vi "Barkod Tarayici.vi"() -> ()   [LabVIEW 2017]
uses:
  <vilib>/userdefined/High Color/IMAQdx.ctl
  <vilib>/Utility/file.llb/Read Delimited Spreadsheet (string).vi
  <vilib>/vision/driver/NI_Vision_Acquisition_Software.lvlib
  <vilib>/vision/NI_Vision_Development_Module.lvlib
panel:
  out "Kullanım":string[](array[string])
  out "İlaç İsmi":string[](array[string])
  out "Barkod":string[](array[string])
  out "all rows":string[][](array[string])
  in  "İlaç Listesi":path
  in  "Listeyi Yükle":bool
  out "İlaç Bilgisi":string
  out "Barkod Bulundu":bool
  out "error out 3":errorcluster
  out "Barkod Numarası":string
  in  "Aranacak Barkod Türleri":u32[](array[ring])=[6, 4] items=["Reserved", "Codabar", "Code 39", "Code 93", "Code 128", "EAN 8", "EAN 13", "Interleaved 2 of 5", "MSI", "UPCA", "Pharmacode", "RSS Limited"]
  out "error out 2":errorcluster
  out "error out":errorcluster
  out "Barkod":T1(array[cluster]) {"Confidence Level" format="%.2f"; "Barcode Type" items=["Reserved", "Codabar", "Code 39", "Code 93", "Code 128", "EAN 8", "EAN 13", "Interleaved 2 of 5", "MSI", "UPCA", "Pharmacode", "RSS Limited"]; "Bounding Box"."y" format="%.2f"; "Bounding Box"."x" format="%.2f"}
  out "Görüntü":T2(plugin-control)
  in  "Durdur":bool
  in  "Kamera Kaynağı Seçiniz":T3
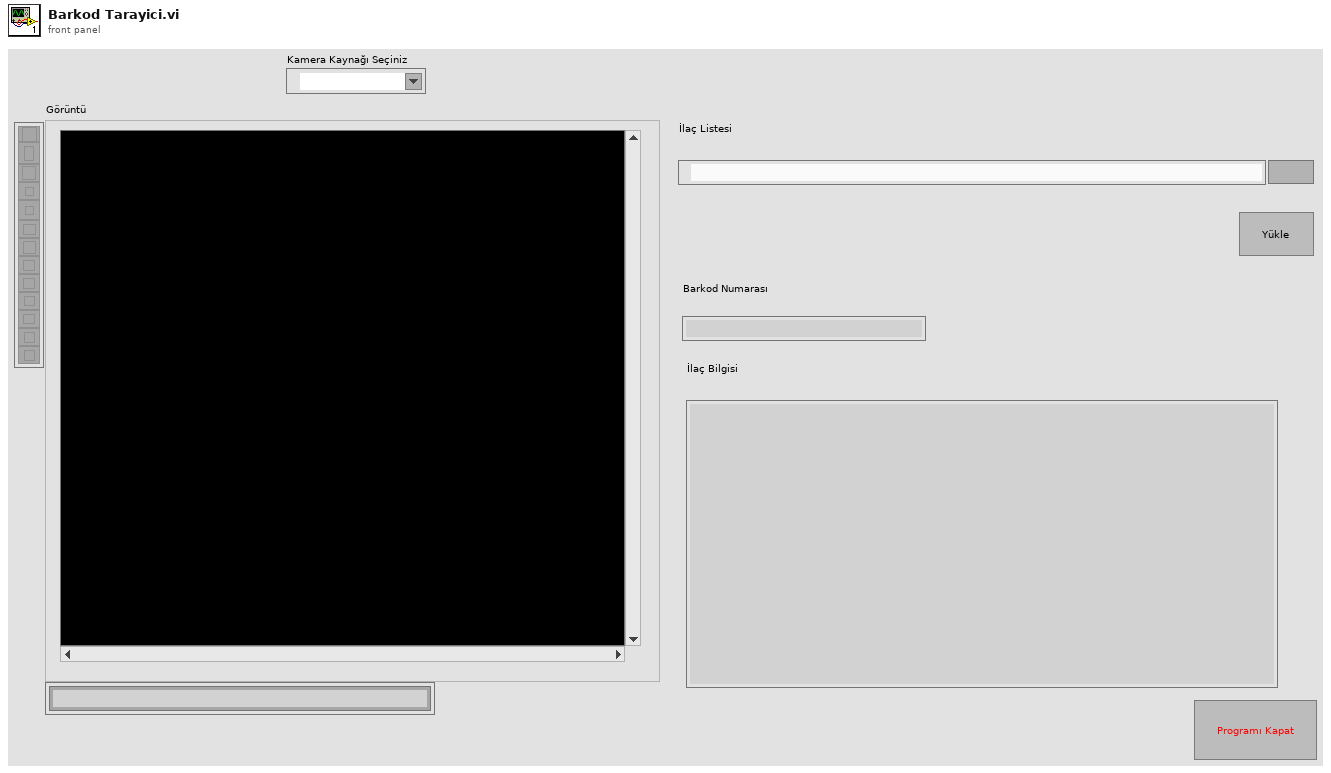
[diagram p1: front panel]
types:
  T1 = cluster{"Data":string, "Special Char 1":string, "Special Char 2":string, "Checksum(s)":string, "Barcode Type":u32, "Confidence Level":sgl, "Bounding Box":cluster{"x":sgl, "y":sgl}[]}[]
  T2 = typedef "IMAQ Image.ctl" = refnum<image>
  T3 = typedef "IMAQdx.ctl" = refnum<k21>
  T4 = cluster{"Data":string, "Special Char 1":string, "Special Char 2":string, "Checksum(s)":string, "Barcode Type":u32, "Confidence Level":sgl, "Bounding Box":cluster{"x":sgl, "y":sgl}[]}
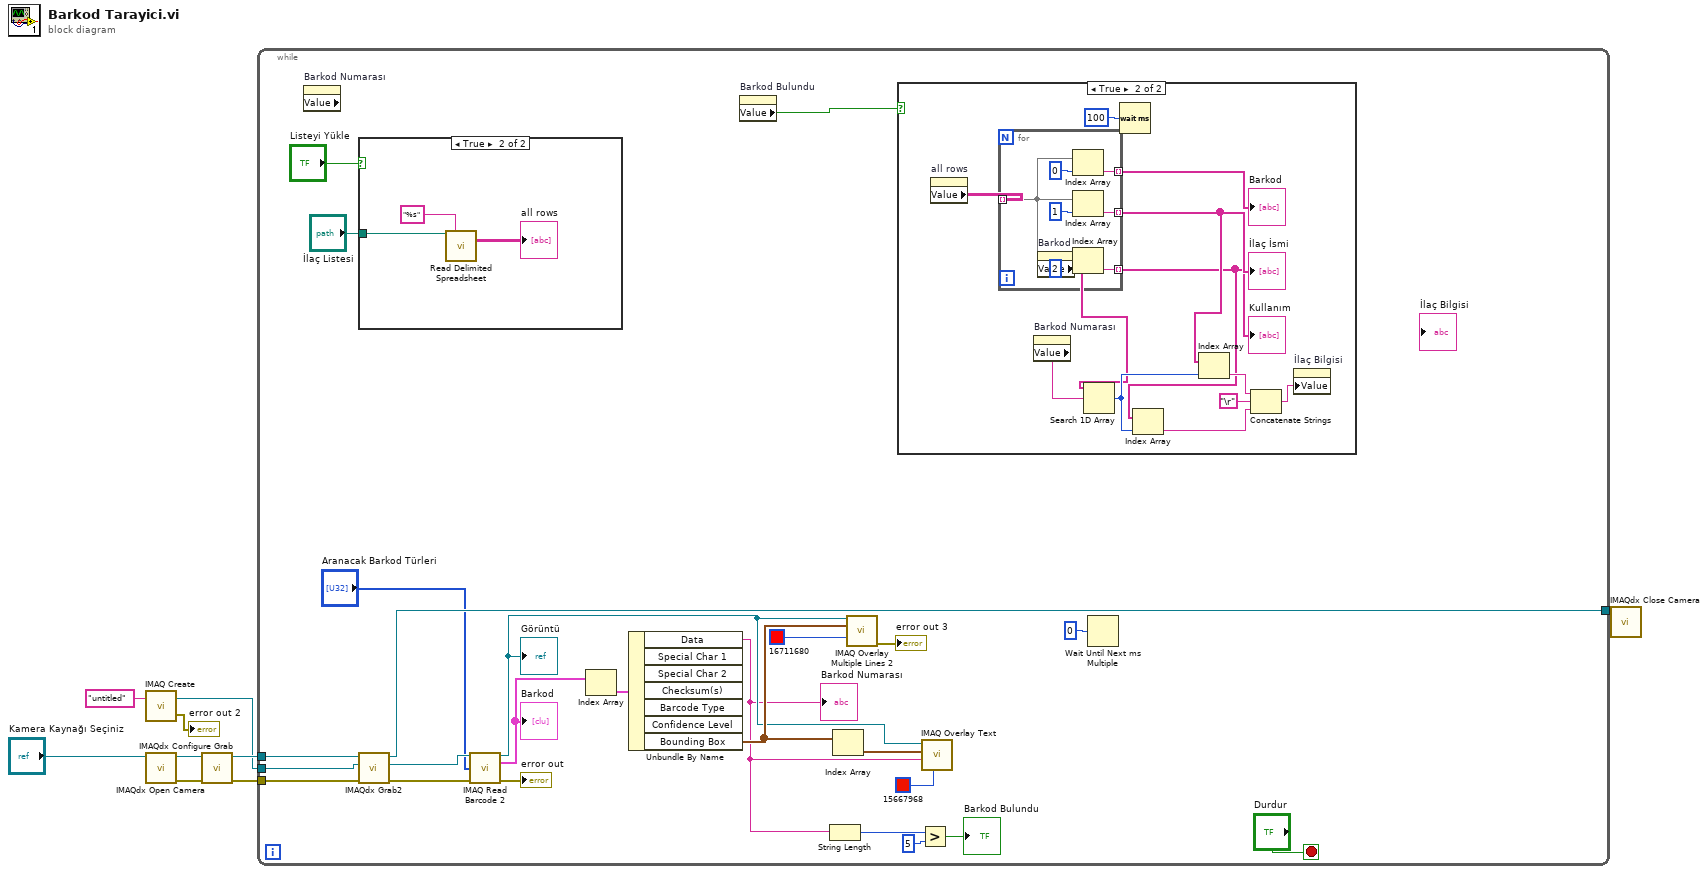
[diagram p0: block diagram]
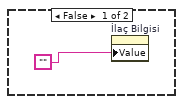
[diagram p3: hidden frame]
diagram:
  n1 = call "IMAQ Create"("Image Name"="untitled") -> ("New Image"=w3:T2, "error out"=→"error out 2":errorcluster)  [unwired: 4 in]
  n2 = call <vilib>:"IMAQdx Open Camera.vi"("Session In"="Kamera Kaynağı Seçiniz") -> ("error out"=w8:errorcluster, "Session Out"=w9:T3)  [unwired: 9 in]
  n3 = call <vilib>:"IMAQdx Configure Grab.vi"("error in"=w8, "Session In"=w9) -> ("error out"=w2:errorcluster, "Session Out"=w7:T3)  [unwired: 8 in]
  n4 = while {
    tunnel: w7 -> [w34]
    tunnel: [w33] -> w6
    tunnel: w3 -> [w31]
    tunnel: w2 -> [w29]
    stop <- "Durdur" stop-if-true
    n5 = property on="Barkod Numarası" class="Str" props=["Value"]() -> ()  [unwired: 2 in, 3 out]
    n6 = case shown="True" "Listeyi Yükle" {
      tunnel: "İlaç Listesi" -> [_ w35]
      frame False {
      }
      frame True {
        n7 = call-poly <vilib>:"Read Delimited Spreadsheet.vi"("file path (dialog if empty)"=w35, "format (%s)"="%s") -> ("all rows"=→"all rows":string[][])  [unwired: 8 in, 5 out]
      }
    }
    n8 = call <vilib>:"IMAQdx Grab2.vi"("error in"=w29, "Image In"=w31, "Session In"=w34) -> ("error out"=w28:errorcluster, "Image Out"=w30:T2, "Session Out"=w33:T3)  [unwired: 5 in, 1 out]
    n9 = call "IMAQ Read Barcode 2"("Image"=w30, "Barcode Types To Search"="Aranacak Barkod Türleri", "error in (no error)"=w28) -> ("Image (duplicate)"=w18:T2, "Barcodes"=w25:T1, "error out"=→"error out":errorcluster)  [unwired: 8 in, 2 out]
    "Görüntü" <- w18
    "Barkod" <- w25
    n10 = Index Array(array=w25) -> (element=w24:T4)  [unwired: 1 in]
    n11 = Unbundle By Name(w24) -> ("Data"=w16:string, "Bounding Box"=w20:cluster{"x":sgl, "y":sgl}[])  [unwired: 5 out]
    "Barkod Numarası" <- w16
    n12 = property on="Barkod Bulundu" class="Bool (strict)"() -> ("Value"=w12:bool)  [unwired: 2 in, 2 out]
    n13 = String Length(string=w16) -> (length=w15:i32)
    n14 = Index Array(array=w20) -> (element=w23:cluster{"x":sgl, "y":sgl})  [unwired: 1 in]
    n15 = call "IMAQ Overlay Multiple Lines 2"("Image"=w18, "Line End Points"=w20, "Color"=u32 16711680) -> ("error out"=→"error out 3":errorcluster)  [unwired: 11 in, 1 out]
    n16 = case shown="True" w12 {
      frame False {
        n17 = property on="İlaç Bilgisi" class="Str"("Value"="") -> ()  [unwired: 2 in, 2 out]
      }
      frame True {
        n18 = property on="all rows" class="Arr (strict)"() -> ("Value"=w42:string[][])  [unwired: 2 in, 2 out]
        n19 = for {
          tunnel: w42 -> [w53] mode=indexing
          tunnel: [w57] -> w43 mode=indexing
          tunnel: [w54] -> w41 mode=indexing
          tunnel: [w51] -> w40 mode=indexing
          n20 = Index Array(array=w53, index=0) -> (element=w57:string)
          n21 = Index Array(array=w53, index=1) -> (element=w54:string)
          n22 = Index Array(array=w53, index=2) -> (element=w51:string)
        }
        "Barkod" <- w43
        "İlaç İsmi" <- w41
        "Kullanım" <- w40
        n23 = property on="Barkod Numarası" class="Str"() -> ("Value"=w44:string)  [unwired: 2 in, 2 out]
        n24 = property on="Barkod" class="Arr (strict)"() -> ("Value"=w45:string[])  [unwired: 2 in, 2 out]
        n25 = Search 1D Array(1D array=w45, element=w44) -> (index of element=w46:i32)  [unwired: 1 in]
        n26 = Wait (ms)(milliseconds to wait=u32 100) -> ()  [unwired: 1 out]
        n27 = Index Array(array=w40, index=w46) -> (element=w47:string)
        n28 = Index Array(array=w41, index=w46) -> (element=w49:string)
        n29 = Concatenate Strings(w49, "\r", w47) -> (w39:string)
        n30 = property on="İlaç Bilgisi" class="Str"("Value"=w39) -> ()  [unwired: 2 in, 2 out]
      }
    }
    n31 = Greater?(x=w15, y=5) -> (0:→"Barkod Bulundu":bool)
    n32 = call "IMAQ Overlay Text"("Text Color (black)"=u32 15667968, "String"=w16, "Origin"=w23, "Image"=w18) -> ()  [unwired: 6 in, 2 out]
    n33 = Wait Until Next ms Multiple(millisecond multiple=u32 0) -> ()  [unwired: 1 out]
  }
  n34 = call <vilib>:"IMAQdx Close Camera.vi"("Session In"=w6) -> ()  [unwired: 10 in, 1 out]
